vi "Resample Pair of Arrays (single shot).vi"(0 "XY-data in":cluster{"X-array":dbl[], "Y-array":dbl[]} {"Y-array" format="%.2p"; "X-array" format="%.2p"}, 5 "dt":dbl=1.0 format="%.2p", 7 "t0":dbl=-inf format="%.2p", 9 "interpolation mode":u16(ring)=1 items=["coerce", "linear", "spline", "FIR filter"], 11 "error in (no error)":errorcluster) -> (4 "resampled waveform out":waveform(dbl), 6 "XY-data out":cluster{"X-array":dbl[], "Y-array":dbl[]} {"Y-array" format="%.2p"; "X-array" format="%.2p"}, 10 "used t0":dbl format="%.2p", 14 "t0 adjusted warning":bool, 15 "error out":errorcluster)   [LabVIEW 2020, in "NI_MAPro.lvlib"]
doc: "Resamples input waveforms or data according to the user-defined <B>t0</B> and <B>dt</B> values.\n\nWire data to the waveform or data input to determine the polymorphic instance to use or manually select the instance."
uses:
  NI_MAPro.lvlib
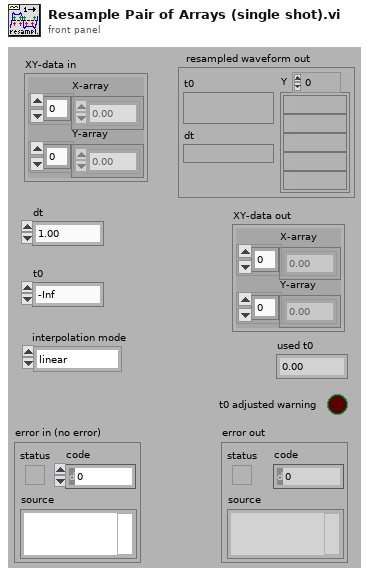
[diagram p1: front panel]
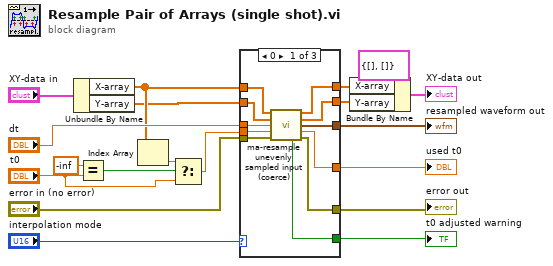
[diagram p0: block diagram]
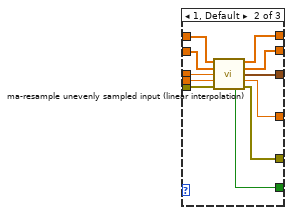
[diagram p2: hidden frame]
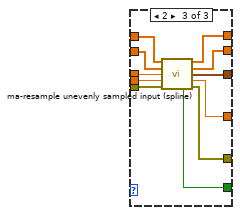
[diagram p3: hidden frame]
diagram:
  n1 = Unbundle By Name("XY-data in") -> ("X-array"=w7:dbl[], "Y-array"=w6:dbl[])
  n2 = Equal?(x=-inf, y="t0") -> (x = y?=w17:bool)
  n3 = Index Array(array=w7) -> (element=w9:dbl)  [unwired: 1 in]
  n4 = Select(t=w9, s=w17, f="t0") -> (s? t:f=w15:dbl)
  n5 = case shown="0" "interpolation mode" {
    tunnel: "error in (no error)" -> [w30 w41 w52]
    tunnel: "dt" -> [w29 w40 w51]
    tunnel: w15 -> [w28 w39 w50]
    tunnel: [w27 w38 w49] -> w14
    tunnel: [w26 w37 w48] -> w13
    tunnel: [w25 w36 w47] -> w12
    tunnel: [w24 w35 w46] -> w11
    tunnel: w7 -> [w21 w34 w43]
    tunnel: w6 -> [w20 w33 w42]
    tunnel: [w23 w32 w45] -> w3
    tunnel: [w22 w31 w44] -> w4
    frame 0 {
      n6 = call "ma-resample unevenly sampled input (coerce).vi"("X-array in"=w21, "Y-array in"=w20, "dt"=w29, "t0"=w28, "error in"=w30) -> ("X-array out"=w22:dbl[], "Y-array out"=w23:dbl[], "evenly sampled waveform out"=w24:waveform(dbl), "used t0"=w25:dbl, "t0 adjusted warning"=w27:bool, "error out"=w26:errorcluster)  [unwired: 5 in]
    }
    frame 1, Default {
      n7 = call "ma-resample unevenly sampled input (linear interpolation).vi"("X-array in"=w34, "Y-array in"=w33, "dt"=w40, "t0"=w39, "error in"=w41) -> ("X-array out"=w31:dbl[], "Y-array out"=w32:dbl[], "evenly sampled waveform out"=w35:waveform(dbl), "used t0"=w36:dbl, "t0 adjusted warning"=w38:bool, "error out"=w37:errorcluster)  [unwired: 5 in]
    }
    frame 2 {
      n8 = call "ma-resample unevenly sampled input (spline).vi"("X-array in"=w43, "Y-array in"=w42, "dt"=w51, "t0"=w50, "error in"=w52) -> ("X-array out"=w44:dbl[], "Y-array out"=w45:dbl[], "evenly sampled waveform out"=w46:waveform(dbl), "used t0"=w47:dbl, "t0 adjusted warning"=w49:bool, "error out"=w48:errorcluster)  [unwired: 5 in]
    }
  }
  "error out" <- w13
  "t0 adjusted warning" <- w14
  "used t0" <- w12
  "resampled waveform out" <- w11
  n9 = Bundle By Name(cluster=cluster{"X-array":dbl[], "Y-array":dbl[]} {"X-array"=[], "Y-array"=[]} ("XY-data out"), "X-array"=w4, "Y-array"=w3) -> (→"XY-data out":cluster{"X-array":dbl[], "Y-array":dbl[]})
